vi "ProcessDigitalTachometer.vi"(7 "Tachometer in":T1, 8 "error in (no error)":errorcluster, 10 "OS Clk Start":dbl, 11 "pulses":dbl[](array[numeric])) -> (0 "error out":errorcluster, 2 "Instant RPM":dbl, 3 "speed position info":T4, 5 "Tachometer out":T1)   [LabVIEW 2017, in "CmsVirtualChannel.lvlib"]
uses:
  <vilib>/addons/InsightCM/Devices/Shared/Cms/CmsVirtualChannel/CmsVirtualChannel.lvlib
  <vilib>/addons/Sound and Vibration/Order Analysis/Misc/OAT Position Info.ctl
  <vilib>/addons/InsightCM/Devices/Shared/Cms/CmsVirtualChannel/controls/Tachometer.ctl
  <vilib>/addons/InsightCM/Utilities/Analysis/Vibration/controls/Tachometer.ctl
  <vilib>/addons/InsightCM/Utilities/Analysis/Vibration/controls/DigitalTachometer.ctl
  <vilib>/addons/InsightCM/Utilities/Analysis/Vibration/VibrationAnalysisFunctions.lvlib
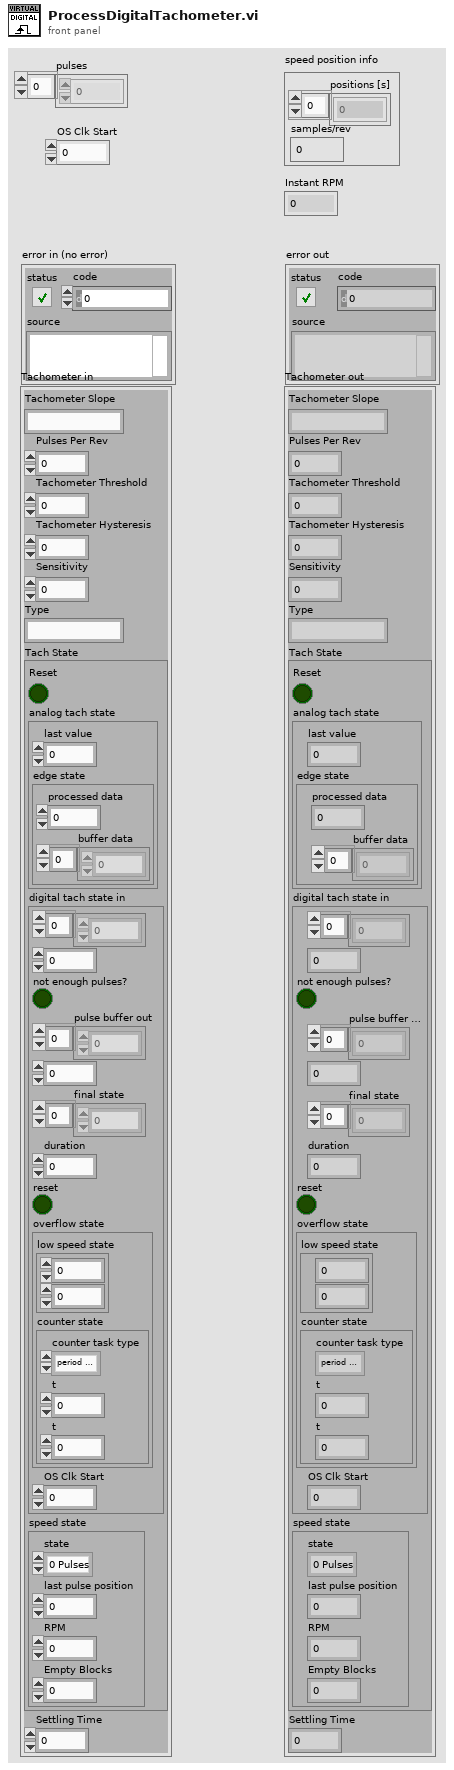
[diagram p1: front panel]
types:
  T1 = typedef "CmsVirtualChannel.lvlib/Tachometer.ctl" = cluster{"Tachometer Slope":string, "Pulses Per Rev":i32, "Tachometer Threshold":dbl, "Tachometer Hysteresis":dbl, "Sensitivity":dbl, "Type":string, "Tach State":T2, "Settling Time":dbl}
  T2 = typedef "VibrationAnalysisFunctions.lvlib/Tachometer.ctl" = cluster{"Reset":bool, "analog tach state":cluster{"last value":dbl, "edge state":cluster{"processed data":dbl, "buffer data":dbl[]}}, "digital tach state in":T3, "speed state":cluster{"state":enum16{"0 Pulses", "1 Pulse", "2+ Pulses"}, "last pulse position":dbl, "RPM":dbl, "Empty Blocks":i32}}
  T3 = typedef "VibrationAnalysisFunctions.lvlib/DigitalTachometer.ctl" = cluster{dbl[], i32, "not enough pulses?":bool, "pulse buffer out":dbl[], i32, "final state":dbl[], "duration":dbl, "reset":bool, "overflow state":cluster{"low speed state":cluster{dbl, ext}, "counter state":cluster{"counter task type":enum16{"period measurement", "event counting"}, "t":dbl, "t":dbl}}, "OS Clk Start":dbl}
  T4 = typedef "OAT Position Info.ctl" = cluster{"positions [s]":dbl[], "samples/rev":dbl}
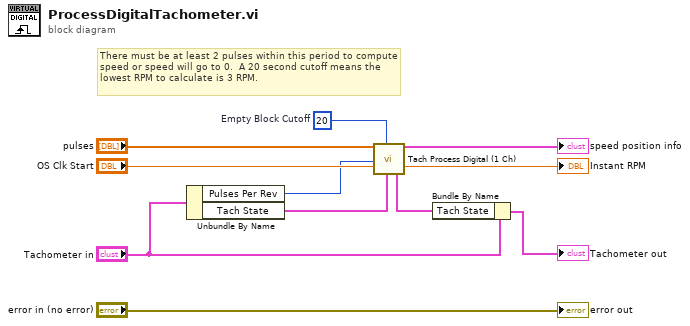
[diagram p0: block diagram]
diagram:
  w8 = 20  # Empty Block Cutoff
  # "There must be at least 2 pulses within this period to compute speed or speed will go to 0.  A 20 second cutoff means the lowest RPM to calculate is 3 RPM."
  n1 = Unbundle By Name("Tachometer in") -> ("Pulses Per Rev"=w4:i32, "Tach State"=w5:T2)
  n2 = call <vilib>:"Tach Process Digital (1 Ch).vi"("digital pulses"="pulses", "pulse/revolution (1)"=w4, "OS Clk Start"="OS Clk Start", "Empty Block Cutoff"=w8, "tach state in"=w5) -> ("tach state out"=w2:T2, "speed position info"=→"speed position info":T4, "Instant RPM"=→"Instant RPM":dbl)  [unwired: 12 in]
  n3 = Bundle By Name(cluster="Tachometer in", "Tach State"=w2) -> (→"Tachometer out":T1)
  "error out" <- "error in (no error)"
